vi "open.vi"(8 "error in (no error)":errorcluster, 11 "Instrument in":refnum<class "Picomotor.lvclass">) -> (0 "error out":errorcluster, 3 "Instrument out":refnum<class "Picomotor.lvclass">)   [LabVIEW 2020, in "Picomotor.lvclass"]
uses:
  Picomotor.lvclass
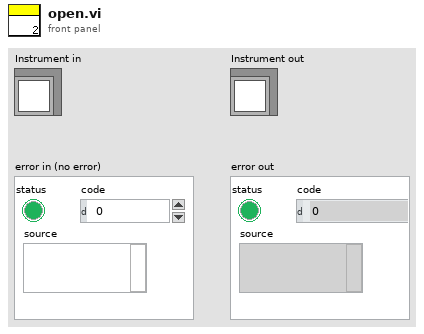
[diagram p1: front panel]
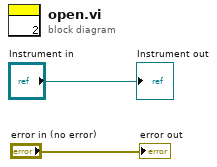
[diagram p0: block diagram]
diagram:
  "error out" <- "error in (no error)"
  "Instrument out" <- "Instrument in"
